vi "q2 count threshold.vi"() -> ()   [LabVIEW 2025]
panel:
  in  "Array":dbl[](array[numeric])
  out "count":dbl
  in  "threshold":dbl
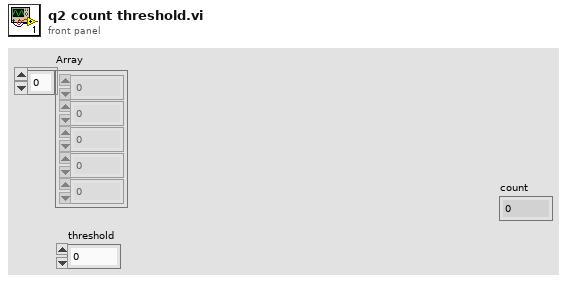
[diagram p1: front panel]
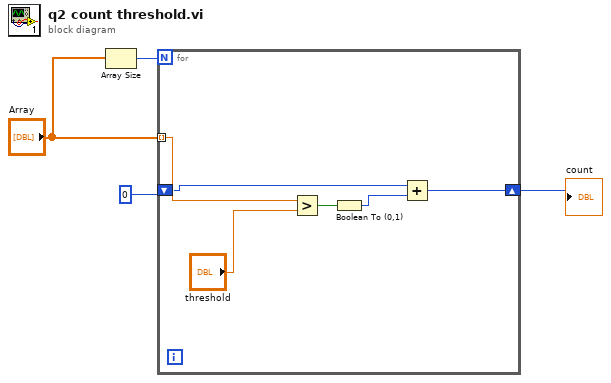
[diagram p0: block diagram]
diagram:
  n1 = Array Size(array="Array") -> (size(s)=w4:i32)
  n2 = for {
    N: w4 -> [_]
    tunnel: "Array" -> [w10] mode=indexing
    shift-right: [w5] -> w1
    shift-left: 0 -> [w6]
    n3 = Greater?(x=w10, y="threshold") -> (0:w8:bool)
    n4 = Boolean To (0,1)(Boolean=w8) -> (0, 1=w7:i16)
    n5 = Add(x=w6, y=w7) -> (x+y=w5:i32)
  }
  "count" <- w1
